vi "Get Parent Message Class Path.vi"(8 "error in (no error)":errorcluster, 11 "Message Scripter in":refnum<class "Message Scripter.lvclass">) -> (0 "error out":errorcluster, 2 "Parent Message":path)   [LabVIEW 2020, in "Message Maker.lvlib" / "Message Scripter.lvclass"]
uses:
  Message Scripter.lvclass
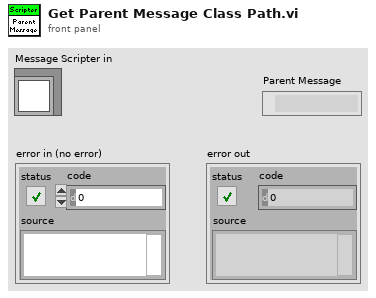
[diagram p1: front panel]
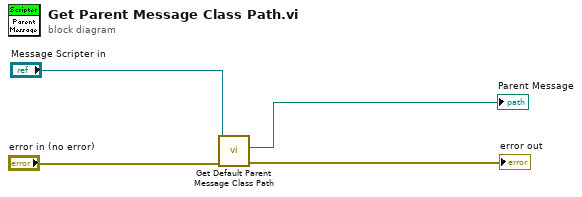
[diagram p0: block diagram]
diagram:
  n1 = call "Get Default Parent Message Class Path.vi"("error in (no error)"="error in (no error)", "Message Scripter"="Message Scripter in") -> ("error out"=→"error out":errorcluster, "Path String"=→"Parent Message":path)  [unwired: 8 in]
